vi "Target Detect HS from GRF.vi"(6 "Sampling Frequency (Hz)":dbl, 8 "HS Threshold":dbl, 9 "LP Filter Cutoff\nFrequency":dbl=12.0 format="%#_13g", 10 "Saturation Threshold":dbl, 11 "Fz":dbl) -> (0 "HS":bool, 3 "GRF Rate (N/s)":dbl, 5 "Filtered Fz":dbl format="%0.2f")   [LabVIEW 2018, in "COBRA Gait Phase Estimation Library.lvlib"]
uses:
  COBRA Gait Phase Estimation Library.lvlib
  <vilib>/Analysis/3filter.llb/Filter Passband Type.ctl
  <vilib>/ptbypt/NI_PtbyPt.lvlib
  <vilib>/Analysis/NI_AALBase.lvlib
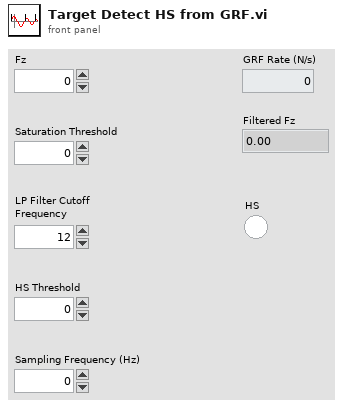
[diagram p1: front panel]
types:
  T1 = typedef "NI_AALBase.lvlib/Filter Passband Type.ctl" = enum32{"Lowpass", "Highpass", "Bandpass", "Bandstop"}
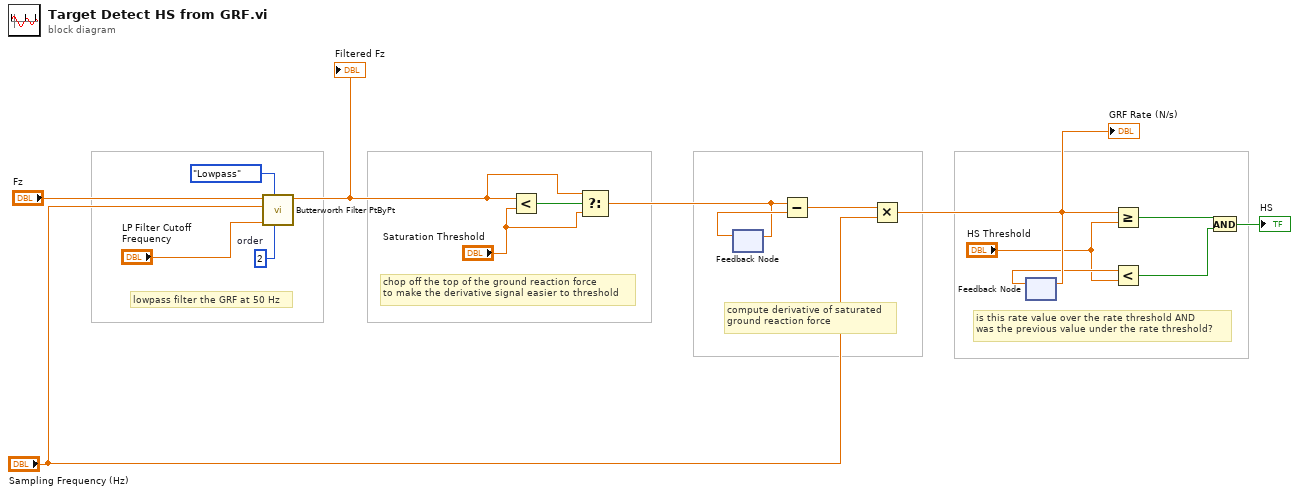
[diagram p0: block diagram]
diagram:
  w4 = 2  # order
  # "lowpass filter the GRF at 50 Hz"
  # "chop off the top of the ground reaction force\nto make the derivative signal easier to threshold"
  # "compute derivative of saturated\nground reaction force"
  # "is this rate value over the rate threshold AND\nwas the previous value under the rate threshold?"
  n1 = call <vilib>:"Butterworth Filter PtByPt.vi"("order"=w4, "filter type"=Filter_Passband_Type."Lowpass", "low cutoff freq: fl"="LP Filter Cutoff\nFrequency", "sampling freq: fs"="Sampling Frequency (Hz)", "x"="Fz") -> ("Filtered x"=w2:dbl)  [unwired: 4 in, 1 out]
  "Filtered Fz" <- w2
  n2 = Less?(x=w2, y="Saturation Threshold") -> (x < y?=w9:bool)
  n3 = Select(t=w2, s=w9, f="Saturation Threshold") -> (s? t:f=w7:dbl)
  n4 = feedback-in #1(w7) -> ()
  n5 = feedback #1() -> (w17:dbl)  [unwired: 1 in]
  n6 = Subtract(x=w7, y=w17) -> (x-y=w16:dbl)
  n7 = Multiply(x=w16, y="Sampling Frequency (Hz)") -> (x*y=w14:dbl)
  "GRF Rate (N/s)" <- w14
  n8 = feedback-in #2(w14) -> ()
  n9 = feedback #2() -> (w13:dbl)  [unwired: 1 in]
  n10 = Greater Or Equal?(x=w14, y="HS Threshold") -> (x >= y?=w12:bool)
  n11 = Less?(x=w13, y="HS Threshold") -> (x < y?=w11:bool)
  n12 = And(x=w12, y=w11) -> (x .and. y?=→"HS":bool)
